vi "rsidr_core_global.vi"() -> ()   [LabVIEW 2015, in "Rohde&Schwarz CMXP NR FR2 Measurement.lvlib"] (continued)
s955, s956, s957, s958, s959, s960, s961, s962, s963, s964, s965, s966, s967, s968, s969, s970, s971, s972, s973, s974, s975, s976, s977, s978, s979, s980, s981, s982, s983, s984, s985, s986, s987, s988, s989, s990, s991, s992, s993, s994, s995, s996, s997, s998, s999, s1000\r\n\nRemote-control command(s):\nCONFigure:NRMMw:MEAS<i>:LIST:SEGMent<no>:SEMask"}, {"Level"=4, "Class Only"=FALSE, "Identifier"="RSCMXPNRFR2M_ATTR_MULTI_EVAL_MEASUREMENT_LIST_SEGMENT_ACLR", "Descriptive Name"="Multi Eval Measurement List Segment ACLR", "Data Type"=enum."RawString", "Command"="CONF:NRMM:MEAS{instance}:LIST:SEGM{Segment}:ACLR", "Access"=enum."Read/Write", "Range Table"="", "Read Callback"="", "Write Callback"="", "Range Callback"="", "Check Callback"="", "Rngtable Callback"="", "Coerce Callback"="", "Supported Models"="", "Instrument Options"="", "Check Status Callback"="", "Flags"=0, "Help"="Defines settings for ACLR measurements in list mode for segment <no>.\n\nSyntax:\nCONFigure:NRMMw:MEAS<i>:LIST:SEGMent<no>:ACLR <ACLRstatistics>, <ACLRenable>\n\n<ACLRstatistics>\nStatistical length in slots\ninteger\nValid Values: 1 to 1000\n \n<ACLRenable>\nEnable or disable the measurement of ACLR results\nValid Values:\nOFF\nON\n\nAvailable Repeated Capabilities:\ninstance: i0, i1, i2, i3, i4, i5, i6, i7, i8, i9, i10, i11, i12, i13, i14, i15, i16, i17, i18, i19, i20, i21, i22, i23, i24, i25, i26, i27, i28, i29, i30, i31, i32\r\nSegment: s1, s2, s3, s4, s5, s6, s7, s8, s9, s10, s11, s12, s13, s14, s15, s16, s17, s18, s19, s20, s21, s22, s23, s24, s25, s26, s27, s28, s29, s30, s31, s32, s33, s34, s35, s36, s37, s38, s39, s40, s41, s42, s43, s44, s45, s46, s47, s48, s49, s50, s51, s52, s53, s54, s55, s56, s57, s58, s59, s60, s61, s62, s63, s64, s65, s66, s67, s68, s69, s70, s71, s72, s73, s74, s75, s76, s77, s78, s79, s80, s81, s82, s83, s84, s85, s86, s87, s88, s89, s90, s91, s92, s93, s94, s95, s96, s97, s98, s99, s100, s101, s102, s103, s104, s105, s106, s107, s108, s109, s110, s111, s112, s113, s114, s115, s116, s117, s118, s119, s120, s121, s122, s123, s124, s125, s126, s127, s128, s129, s130, s131, s132, s133, s134, s135, s136, s137, s138, s139, s140, s141, s142, s143, s144, s145, s146, s147, s148, s149, s150, s151, s152, s153, s154, s155, s156, s157, s158, s159, s160, s161, s162, s163, s164, s165, s166, s167, s168, s169, s170, s171, s172, s173, s174, s175, s176, s177, s178, s179, s180, s181, s182, s183, s184, s185, s186, s187, s188, s189, s190, s191, s192, s193, s194, s195, s196, s197, s198, s199, s200, s201, s202, s203, s204, s205, s206, s207, s208, s209, s210, s211, s212, s213, s214, s215, s216, s217, s218, s219, s220, s221, s222, s223, s224, s225, s226, s227, s228, s229, s230, s231, s232, s233, s234, s235, s236, s237, s238, s239, s240, s241, s242, s243, s244, s245, s246, s247, s248, s249, s250, s251, s252, s253, s254, s255, s256, s257, s258, s259, s260, s261, s262, s263, s264, s265, s266, s267, s268, s269, s270, s271, s272, s273, s274, s275, s276, s277, s278, s279, s280, s281, s282, s283, s284, s285, s286, s287, s288, s289, s290, s291, s292, s293, s294, s295, s296, s297, s298, s299, s300, s301, s302, s303, s304, s305, s306, s307, s308, s309, s310, s311, s312, s313, s314, s315, s316, s317, s318, s319, s320, s321, s322, s323, s324, s325, s326, s327, s328, s329, s330, s331, s332, s333, s334, s335, s336, s337, s338, s339, s340, s341, s342, s343, s344, s345, s346, s347, s348, s349, s350, s351, s352, s353, s354, s355, s356, s357, s358, s359, s360, s361, s362, s363, s364, s365, s366, s367, s368, s369, s370, s371, s372, s373, s374, s375, s376, s377, s378, s379, s380, s381, s382, s383, s384, s385, s386, s387, s388, s389, s390, s391, s392, s393, s394, s395, s396, s397, s398, s399, s400, s401, s402, s403, s404, s405, s406, s407, s408, s409, s410, s411, s412, s413, s414, s415, s416, s417, s418, s419, s420, s421, s422, s423, s424, s425, s426, s427, s428, s429, s430, s431, s432, s433, s434, s435, s436, s437, s438, s439, s440, s441, s442, s443, s444, s445, s446, s447, s448, s449, s450, s451, s452, s453, s454, s455, s456, s457, s458, s459, s460, s461, s462, s463, s464, s465, s466, s467, s468, s469, s470, s471, s472, s473, s474, s475, s476, s477, s478, s479, s480, s481, s482, s483, s484, s485, s486, s487, s488, s489, s490, s491, s492, s493, s494, s495, s496, s497, s498, s499, s500, s501, s502, s503, s504, s505, s506, s507, s508, s509, s510, s511, s512, s513, s514, s515, s516, s517, s518, s519, s520, s521, s522, s523, s524, s525, s526, s527, s528, s529, s530, s531, s532, s533, s534, s535, s536, s537, s538, s539, s540, s541, s542, s543, s544, s545, s546, s547, s548, s549, s550, s551, s552, s553, s554, s555, s556, s557, s558, s559, s560, s561, s562, s563, s564, s565, s566, s567, s568, s569, s570, s571, s572, s573, s574, s575, s576, s577, s578, s579, s580, s581, s582, s583, s584, s585, s586, s587, s588, s589, s590, s591, s592, s593, s594, s595, s596, s597, s598, s599, s600, s601, s602, s603, s604, s605, s606, s607, s608, s609, s610, s611, s612, s613, s614, s615, s616, s617, s618, s619, s620, s621, s622, s623, s624, s625, s626, s627, s628, s629, s630, s631, s632, s633, s634, s635, s636, s637, s638, s639, s640, s641, s642, s643, s644, s645, s646, s647, s648, s649, s650, s651, s652, s653, s654, s655, s656, s657, s658, s659, s660, s661, s662, s663, s664, s665, s666, s667, s668, s669, s670, s671, s672, s673, s674, s675, s676, s677, s678, s679, s680, s681, s682, s683, s684, s685, s686, s687, s688, s689, s690, s691, s692, s693, s694, s695, s696, s697, s698, s699, s700, s701, s702, s703, s704, s705, s706, s707, s708, s709, s710, s711, s712, s713, s714, s715, s716, s717, s718, s719, s720, s721, s722, s723, s724, s725, s726, s727, s728, s729, s730, s731, s732, s733, s734, s735, s736, s737, s738, s739, s740, s741, s742, s743, s744, s745, s746, s747, s748, s749, s750, s751, s752, s753, s754, s755, s756, s757, s758, s759, s760, s761, s762, s763, s764, s765, s766, s767, s768, s769, s770, s771, s772, s773, s774, s775, s776, s777, s778, s779, s780, s781, s782, s783, s784, s785, s786, s787, s788, s789, s790, s791, s792, s793, s794, s795, s796, s797, s798, s799, s800, s801, s802, s803, s804, s805, s806, s807, s808, s809, s810, s811, s812, s813, s814, s815, s816, s817, s818, s819, s820, s821, s822, s823, s824, s825, s826, s827, s828, s829, s830, s831, s832, s833, s834, s835, s836, s837, s838, s839, s840, s841, s842, s843, s844, s845, s846, s847, s848, s849, s850, s851, s852, s853, s854, s855, s856, s857, s858, s859, s860, s861, s862, s863, s864, s865, s866, s867, s868, s869, s870, s871, s872, s873, s874, s875, s876, s877, s878, s879, s880, s881, s882, s883, s884, s885, s886, s887, s888, s889, s890, s891, s892, s893, s894, s895, s896, s897, s898, s899, s900, s901, s902, s903, s904, s905, s906, s907, s908, s909, s910, s911, s912, s913, s914, s915, s916, s917, s918, s919, s920, s921, s922, s923, s924, s925, s926, s927, s928, s929, s930, s931, s932, s933, s934, s935, s936, s937, s938, s939, s940, s941, s942, s943, s944, s945, s946, s947, s948, s949, s950, s951, s952, s953, s954, s955, s956, s957, s958, s959, s960, s961, s962, s963, s964, s965, s966, s967, s968, s969, s970, s971, s972, s973, s974, s975, s976, s977, s978, s979, s980, s981, s982, s983, s984, s985, s986, s987, s988, s989, s990, s991, s992, s993, s994, s995, s996, s997, s998, s999, s1000\r\n\nRemote-control command(s):\nCONFigure:NRMMw:MEAS<i>:LIST:SEGMent<no>:ACLR"}, {"Level"=2, "Class Only"=TRUE, "Identifier"="", "Descriptive Name"="Trigger", "Data Type"=enum."ViInt32", "Command"="", "Access"=enum."Read Only", "Range Table"="", "Read Callback"="", "Write Callback"="", "Range Callback"="", "Check Callback"="", "Rngtable Callback"="", "Coerce Callback"="", "Supported Models"="", "Instrument Options"="", "Check Status Callback"="", "Flags"=0, "Help"="Trigger settings"}, {"Level"=3, "Class Only"=FALSE, "Identifier"="RSCMXPNRFR2M_ATTR_MULTI_EVAL_MEASUREMENT_TRIGGER_SOURCE", "Descriptive Name"="Multi Eval Measurement Trigger Source", "Data Type"=enum."ViString", "Command"="TRIG:NRMM:MEAS{instance}:MEV:SOUR", "Access"=enum."Read/Write", "Range Table"="", "Read Callback"="", "Write Callback"="", "Range Callback"="", "Check Callback"="", "Rngtable Callback"="", "Coerce Callback"="", "Supported Models"="", "Instrument Options"="", "Check Status Callback"="", "Flags"=0, "Help"="Selects the source of the trigger events. Some values are always available. You can query a list of all supported values via TRIGger:...:CATalog:SOURce?\n\nAvailable Repeated Capabilities:\ninstance: i0, i1, i2, i3, i4, i5, i6, i7, i8, i9, i10, i11, i12, i13, i14, i15, i16, i17, i18, i19, i20, i21, i22, i23, i24, i25, i26, i27, i28, i29, i30, i31, i32\r\n\nRemote-control command(s):\nTRIGger:NRMMw:MEAS<i>:MEValuation:SOURce"}, {"Level"=3, "Class Only"=FALSE, "Identifier"="RSCMXPNRFR2M_ATTR_MULTI_EVAL_MEASUREMENT_TRIGGER_SOURCE_CATALOG", "Descriptive Name"="Multi Eval Measurement Trigger Source Catalog", "Data Type"=enum."RawString", "Command"="TRIG:NRMM:MEAS{instance}:MEV:CAT:SOUR?", "Access"=enum."Read Only", "Range Table"="", "Read Callback"="", "Write Callback"="", "Range Callback"="", "Check Callback"="", "Rngtable Callback"="", "Coerce Callback"="", "Supported Models"="", "Instrument Options"="", "Check Status Callback"="", "Flags"=0, "Help"="Lists all trigger source values that can be set using TRIGger:NRMMw:MEAS<i>:MEValuation:SOURce. Comma-separated list of all supported values, one string per value.\n\nAvailable Repeated Capabilities:\ninstance: i0, i1, i2, i3, i4, i5, i6, i7, i8, i9, i10, i11, i12, i13, i14, i15, i16, i17, i18, i19, i20, i21, i22, i23, i24, i25, i26, i27, i28, i29, i30, i31, i32\r\n\nRemote-control command(s):\nTRIGger:NRMMw:MEAS<i>:MEValuation:CATalog:SOURce?"}, {"Level"=3, "Class Only"=FALSE, "Identifier"="RSCMXPNRFR2M_ATTR_MULTI_EVAL_MEASUREMENT_TRIGGER_SLOPE", "Descriptive Name"="Multi Eval Measurement Trigger Slope", "Data Type"=enum."ViInt32", "Command"="TRIG:NRMM:MEAS{instance}:MEV:SLOP", "Access"=enum."Read/Write", "Range Table"="rsCmxpNrFr2M_rngTrigSlope", "Read Callback"="", "Write Callback"="", "Range Callback"="", "Check Callback"="", "Rngtable Callback"="", "Coerce Callback"="", "Supported Models"="", "Instrument Options"="", "Check Status Callback"="", "Flags"=0, "Help"="Qualifies whether the trigger event is generated at the rising or at the falling edge of the trigger pulse (valid for external and power trigger sources).\n\nAvailable Repeated Capabilities:\ninstance: i0, i1, i2, i3, i4, i5, i6, i7, i8, i9, i10, i11, i12, i13, i14, i15, i16, i17, i18, i19, i20, i21, i22, i23, i24, i25, i26, i27, i28, i29, i30, i31, i32\r\n\nRemote-control command(s):\nTRIGger:NRMMw:MEAS<i>:MEValuation:SLOPe"}, {"Level"=3, "Class Only"=FALSE, "Identifier"="RSCMXPNRFR2M_ATTR_MULTI_EVAL_MEASUREMENT_TRIGGER_THRESHOLD", "Descriptive Name"="Multi Eval Measurement Trigger Threshold", "Data Type"=enum."ViReal64", "Command"="TRIG:NRMM:MEAS{instance}:MEV:THR", "Access"=enum."Read/Write", "Range Table"="rsCmxpNrFr2M_rngTrigThreshold", "Read Callback"="", "Write Callback"="", "Range Callback"="", "Check Callback"="", "Rngtable Callback"="", "Coerce Callback"="", "Supported Models"="", "Instrument Options"="", "Check Status Callback"="", "Flags"=0, "Help"="Defines the trigger threshold for power trigger sources.\n\nAvailable Repeated Capabilities:\ninstance: i0, i1, i2, i3, i4, i5, i6, i7, i8, i9, i10, i11, i12, i13, i14, i15, i16, i17, i18, i19, i20, i21, i22, i23, i24, i25, i26, i27, i28, i29, i30, i31, i32\r\n\nRemote-control command(s):\nTRIGger:NRMMw:MEAS<i>:MEValuation:THReshold"}, {"Level"=3, "Class Only"=FALSE, "Identifier"="RSCMXPNRFR2M_ATTR_MULTI_EVAL_MEASUREMENT_TRIGGER_DELAY", "Descriptive Name"="Multi Eval Measurement Trigger Delay", "Data Type"=enum."ViReal64", "Command"="TRIG:NRMM:MEAS{instance}:MEV:DEL", "Access"=enum."Read/Write", "Range Table"="rsCmxpNrFr2M_rngMultiEvalMeasurementTriggerDelay", "Read Callback"="", "Write Callback"="", "Range Callback"="", "Check Callback"="", "Rngtable Callback"="", "Coerce Callback"="", "Supported Models"="", "Instrument Options"="", "Check Status Callback"="", "Flags"=0, "Help"="Defines a time delaying the start of the measurement relative to the trigger event. This setting has no influence on free run measurements.\n\nAvailable Repeated Capabilities:\ninstance: i0, i1, i2, i3, i4, i5, i6, i7, i8, i9, i10, i11, i12, i13, i14, i15, i16, i17, i18, i19, i20, i21, i22, i23, i24, i25, i26, i27, i28, i29, i30, i31, i32\r\n\nRemote-control command(s):\nTRIGger:NRMMw:MEAS<i>:MEValuation:DELay"}, {"Level"=3, "Class Only"=FALSE, "Identifier"="RSCMXPNRFR2M_ATTR_MULTI_EVAL_MEASUREMENT_TRIGGER_TIMEOUT_ENABLED", "Descriptive Name"="Multi Eval Measurement Trigger Timeout Enabled", "Data Type"=enum."ViBoolean", "Command"="TRIG:NRMM:MEAS{instance}:MEV:TOUT", "Access"=enum."Write Only", "Range Table"="", "Read Callback"="", "Write Callback"="", "Range Callback"="", "Check Callback"="", "Rngtable Callback"="", "Coerce Callback"="", "Supported Models"="", "Instrument Options"="", "Check Status Callback"="", "Flags"=0, "Help"="Enables/disables trigger timeout.\n\nAvailable Repeated Capabilities:\ninstance: i0, i1, i2, i3, i4, i5, i6, i7, i8, i9, i10, i11, i12, i13, i14, i15, i16, i17, i18, i19, i20, i21, i22, i23, i24, i25, i26, i27, i28, i29, i30, i31, i32\r\n\nRemote-control command(s):\nTRIGger:NRMMw:MEAS<i>:MEValuation:TOUT"}, {"Level"=3, "Class Only"=FALSE, "Identifier"="RSCMXPNRFR2M_ATTR_MULTI_EVAL_MEASUREMENT_TRIGGER_TIMEOUT", "Descriptive Name"="Multi Eval Measurement Trigger Timeout", "Data Type"=enum."ViReal64", "Command"="TRIG:NRMM:MEAS{instance}:MEV:TOUT", "Access"=enum."Read/Write", "Range Table"="rsCmxpNrFr2M_rngTriggerTimeout", "Read Callback"="", "Write Callback"="", "Range Callback"="", "Check Callback"="", "Rngtable Callback"="", "Coerce Callback"="", "Supported Models"="", "Instrument Options"="", "Check Status Callback"="", "Flags"=0, "Help"="Selects the maximum time that the measurement waits for a trigger event before it stops in remote control mode or indicates a trigger timeout in manual operation mode. This setting has no influence on 'Free Run' measurements.\n\nAvailable Repeated Capabilities:\ninstance: i0, i1, i2, i3, i4, i5, i6, i7, i8, i9, i10, i11, i12, i13, i14, i15, i16, i17, i18, i19, i20, i21, i22, i23, i24, i25, i26, i27, i28, i29, i30, i31, i32\r\n\nRemote-control command(s):\nTRIGger:NRMMw:MEAS<i>:MEValuation:TOUT"}, {"Level"=3, "Class Only"=FALSE, "Identifier"="RSCMXPNRFR2M_ATTR_MULTI_EVAL_MEASUREMENT_MINIMUM_TRIGGER_GAP", "Descriptive Name"="Multi Eval Measurement Minimum Trigger Gap", "Data Type"=enum."ViReal64", "Command"="TRIG:NRMM:MEAS{instance}:MEV:MGAP", "Access"=enum."Read/Write", "Range Table"="rsCmxpNrFr2M_rngMultiEvalMeasurementMinimumTriggerGap", "Read Callback"="", "Write Callback"="", "Range Callback"="", "Check Callback"="", "Rngtable Callback"="", "Coerce Callback"="", "Supported Models"="", "Instrument Options"="", "Check Status Callback"="", "Flags"=0, "Help"="Sets a minimum time during which the IF signal must be below the trigger threshold before the trigger is armed so that an IF power trigger event can be generated.\n\nAvailable Repeated Capabilities:\ninstance: i0, i1, i2, i3, i4, i5, i6, i7, i8, i9, i10, i11, i12, i13, i14, i15, i16, i17, i18, i19, i20, i21, i22, i23, i24, i25, i26, i27, i28, i29, i30, i31, i32\r\n\nRemote-control command(s):\nTRIGger:NRMMw:MEAS<i>:MEValuation:MGAP"}, {"Level"=2, "Class Only"=TRUE, "Identifier"="", "Descriptive Name"="Limits", "Data Type"=enum."ViInt32", "Command"="", "Access"=enum."Read Only", "Range Table"="", "Read Callback"="", "Write Callback"="", "Range Callback"="", "Check Callback"="", "Rngtable Callback"="", "Coerce Callback"="", "Supported Models"="", "Instrument Options"="", "Check Status Callback"="", "Flags"=0, "Help"="Multi Evaluation measurement limits attributes."}, {"Level"=3, "Class Only"=TRUE, "Identifier"="", "Descriptive Name"="Modulation", "Data Type"=enum."ViInt32", "Command"="", "Access"=enum."Read Only", "Range Table"="", "Read Callback"="", "Write Callback"="", "Range Callback"="", "Check Callback"="", "Rngtable Callback"="", "Coerce Callback"="", "Supported Models"="", "Instrument Options"="", "Check Status Callback"="", "Flags"=0, "Help"="Modulation attributes."}, {"Level"=4, "Class Only"=TRUE, "Identifier"="", "Descriptive Name"="Pi/2-BPSK", "Data Type"=enum."ViInt32", "Command"="", "Access"=enum."Read Only", "Range Table"="", "Read Callback"="", "Write Callback"="", "Range Callback"="", "Check Callback"="", "Rngtable Callback"="", "Coerce Callback"="", "Supported Models"="", "Instrument Options"="", "Check Status Callback"="", "Flags"=0, "Help"="Define limits for results which characterize the modulation accuracy of signals with modulation scheme Pi/2-BPSK."}, {"Level"=5, "Class Only"=FALSE, "Identifier"="RSCMXPNRFR2M_ATTR_MULTI_EVAL_MEASUREMENT_LIMIT_PHBPSK_EVM", "Descriptive Name"="Multi Eval Measurement Limit PHBPSK EVM", "Data Type"=enum."RawString", "Command"="CONF:NRMM:MEAS{instance}:MEV:LIM:PHBP:EVM", "Access"=enum."Read/Write", "Range Table"="", "Read Callback"="", "Write Callback"="", "Range Callback"="", "Check Callback"="", "Rngtable Callback"="", "Coerce Callback"="", "Supported Models"="", "Instrument Options"="", "Check Status Callback"="", "Flags"=0, "Help"="Defines upper limits for the RMS and peak values of the error vector magnitude (EVM) for Pi/2-BPSK.\n\nSyntax:\nCONFigure:NRMMw:MEAS<i>:MEValuation:LIMit:PHBPsk:EVMagnitude <RMS>, <Peak>\n\n<RMS>\nnumeric | ON | OFF\nValid Values:\n0 % to 100 %\nOFF\nON\n  \n<Peak>\nnumeric | ON | OFF\nValid Values:\n0 % to 100 %\nOFF\nON\n\nAvailable Repeated Capabilities:\ninstance: i0, i1, i2, i3, i4, i5, i6, i7, i8, i9, i10, i11, i12, i13, i14, i15, i16, i17, i18, i19, i20, i21, i22, i23, i24, i25, i26, i27, i28, i29, i30, i31, i32\r\n\nRemote-control command(s):\nCONFigure:NRMMw:MEAS<i>:MEValuation:LIMit:PHBPsk:EVMagnitude"}, {"Level"=5, "Class Only"=FALSE, "Identifier"="RSCMXPNRFR2M_ATTR_MULTI_EVAL_MEASUREMENT_LIMIT_PHBPSK_MERR", "Descriptive Name"="Multi Eval Measurement Limit PHBPSK MERR", "Data Type"=enum."RawString", "Command"="CONF:NRMM:MEAS{instance}:MEV:LIM:PHBP:MERR", "Access"=enum."Read/Write", "Range Table"="", "Read Callback"="", "Write Callback"="", "Range Callback"="", "Check Callback"="", "Rngtable Callback"="", "Coerce Callback"="", "Supported Models"="", "Instrument Options"="", "Check Status Callback"="", "Flags"=0, "Help"="Defines upper limits for the RMS and peak values of the magnitude error (MERR)  for Pi/2-BPSK.\n\nSyntax:\nCONFigure:NRMMw:MEAS<i>:MEValuation:LIMit:PHBPsk:MERRor <RMS>, <Peak>\n\n<RMS>\nnumeric | ON | OFF\nValid Values:\n0 % to 100 %\nOFF\nON\n  \n<Peak>\nnumeric | ON | OFF\nValid Values:\n0 % to 100 %\nOFF\nON\n\nAvailable Repeated Capabilities:\ninstance: i0, i1, i2, i3, i4, i5, i6, i7, i8, i9, i10, i11, i12, i13, i14, i15, i16, i17, i18, i19, i20, i21, i22, i23, i24, i25, i26, i27, i28, i29, i30, i31, i32\r\n\nRemote-control command(s):\nCONFigure:NRMMw:MEAS<i>:MEValuation:LIMit:PHBPsk:MERRor"}, {"Level"=5, "Class Only"=FALSE, "Identifier"="RSCMXPNRFR2M_ATTR_MULTI_EVAL_MEASUREMENT_LIMIT_PHBPSK_PERR", "Descriptive Name"="Multi Eval Measurement Limit PHBPSK PERR", "Data Type"=enum."RawString", "Command"="CONF:NRMM:MEAS{instance}:MEV:LIM:PHBP:PERR", "Access"=enum."Read/Write", "Range Table"="", "Read Callback"="", "Write Callback"="", "Range Callback"="", "Check Callback"="", "Rngtable Callback"="", "Coerce Callback"="", "Supported Models"="", "Instrument Options"="", "Check Status Callback"="", "Flags"=0, "Help"="Defines upper limits for the RMS and peak values of the phase error (PERR)  for Pi/2-BPSK.\n\nSyntax:\nCONFigure:NRMMw:MEAS<i>:MEValuation:LIMit:PHBPsk:PERRor <RMS>, <Peak>\n\n<RMS>\nnumeric | ON | OFF\nValid Values:\n0 % to 100 %\nOFF\nON\n  \n<Peak>\nnumeric | ON | OFF\nValid Values:\n0 % to 100 %\nOFF\nON\n\nAvailable Repeated Capabilities:\ninstance: i0, i1, i2, i3, i4, i5, i6, i7, i8, i9, i10, i11, i12, i13, i14, i15, i16, i17, i18, i19, i20, i21, i22, i23, i24, i25, i26, i27, i28, i29, i30, i31, i32\r\n\nRemote-control command(s):\nCONFigure:NRMMw:MEAS<i>:MEValuation:LIMit:PHBPsk:PERRor"}, {"Level"=5, "Class Only"=FALSE, "Identifier"="RSCMXPNRFR2M_ATTR_MULTI_EVAL_MEASUREMENT_LIMIT_PHBPSK_FERR", "Descriptive Name"="Multi Eval Measurement Limit PHBPSK FERR", "Data Type"=enum."RawString", "Command"="CONF:NRMM:MEAS{instance}:MEV:LIM:PHBP:FERR", "Access"=enum."Read/Write", "Range Table"="", "Read Callback"="", "Write Callback"="", "Range Callback"="", "Check Callback"="", "Rngtable Callback"="", "Coerce Callback"="", "Supported Models"="", "Instrument Options"="", "Check Status Callback"="", "Flags"=0, "Help"="Defines an upper limit for the carrier frequency error (Pi/2-BPSK modulation).\n\nSyntax:\nCONFigure:NRMMw:MEAS<i>:MEValuation:LIMit:PHBPsk:FERRor <FrequencyError>\n\n<FrequencyError>\nnumeric | ON | OFF\nValid Values:\n0 to 1 ppm\nOFF\nON\n\nAvailable Repeated Capabilities:\ninstance: i0, i1, i2, i3, i4, i5, i6, i7, i8, i9, i10, i11, i12, i13, i14, i15, i16, i17, i18, i19, i20, i21, i22, i23, i24, i25, i26, i27, i28, i29, i30, i31, i32\r\n\nRemote-control command(s):\nCONFigure:NRMMw:MEAS<i>:MEValuation:LIMit:PHBPsk:FERRor"}, {"Level"=5, "Class Only"=FALSE, "Identifier"="RSCMXPNRFR2M_ATTR_MULTI_EVAL_MEASUREMENT_LIMIT_PHBPSK_IQ_OFFSET", "Descriptive Name"="Multi Eval Measurement Limit PHBPSK IQ Offset", "Data Type"=enum."RawString", "Command"="CONF:NRMM:MEAS{instance}:MEV:LIM:PHBP:IQOF", "Access"=enum."Read/Write", "Range Table"="", "Read Callback"="", "Write Callback"="", "Range Callback"="", "Check Callback"="", "Rngtable Callback"="", "Coerce Callback"="", "Supported Models"="", "Instrument Options"="", "Check Status Callback"="", "Flags"=0, "Help"="Defines upper limits for the I/Q origin offset (Pi/2-BPSK modulation). Two different I/Q origin offset limits can be set for two TX power ranges.\n\nSyntax:\nCONFigure:NRMMw:MEAS<i>:MEValuation:LIMit:PHBPsk:IQOFfset <Enable>, <Offset0>, <Offset1>\n\n<Enable>\nValid Values:\nOFF: disables the limit check\nON: enables the limit check\n\n<Offset0>\nI/Q origin offset limit for TX power > 0 dBm\nnumeric\nValid Values: -256 dBc to 256 dBc\n\n<Offset1>\nI/Q origin offset limit for TX power  0 dBm\nnumeric\nValid Values: -256 dBc to 256 dBc\n\nAvailable Repeated Capabilities:\ninstance: i0, i1, i2, i3, i4, i5, i6, i7, i8, i9, i10, i11, i12, i13, i14, i15, i16, i17, i18, i19, i20, i21, i22, i23, i24, i25, i26, i27, i28, i29, i30, i31, i32\r\n\nRemote-control command(s):\nCONFigure:NRMMw:MEAS<i>:MEValuation:LIMit:PHBPsk:IQOFfset"}, {"Level"=5, "Class Only"=FALSE, "Identifier"="RSCMXPNRFR2M_ATTR_MULTI_EVAL_MEASUREMENT_LIMIT_PHBPSK_INBAND_EMISSION", "Descriptive Name"="Multi Eval Measurement Limit PHBPSK Inband Emission", "Data Type"=enum."RawString", "Command"="CONF:NRMM:MEAS{instance}:MEV:LIM:PHBP:IBE", "Access"=enum."Read/Write", "Range Table"="", "Read Callback"="", "Write Callback"="", "Range Callback"="", "Check Callback"="", "Rngtable Callback"="", "Coerce Callback"="", "Supported Models"="", "Instrument Options"="", "Check Status Callback"="", "Flags"=0, "Help"="Defines parameters used for calculation of an upper limit for the inband emission (Pi/2-BPSK modulation).\n\nSyntax:\nCONFigure:NRMMw:MEAS<i>:MEValuation:LIMit:PHBPsk:IQOFfset <Enable>, <Offset0>, <Offset1>\n\n<Enable>\nValid Values:\nOFF: disables the limit check\nON: enables the limit check\n\n<Minimum>\nnumeric\nValid Values: -256 dB to 256 dB\n\n<EVM>\nnumeric\nValid Values: 0 % to 100 %\n\n<RBPower>\nnumeric\nValid Values: -256 dBm to 256 dBm\n\n<IQImageLesser>\nIQ image for low TX power range\nnumeric\nValid Values: -256 dB to 256 dB\n \n<IQImageGreater>\nIQ image for high TX power range\nnumeric\nValid Values: -256 dB  to  256 dB\n\nAvailable Repeated Capabilities:\ninstance: i0, i1, i2, i3, i4, i5, i6, i7, i8, i9, i10, i11, i12, i13, i14, i15, i16, i17, i18, i19, i20, i21, i22, i23, i24, i25, i26, i27, i28, i29, i30, i31, i32\r\n\nRemote-control command(s):\nCONFigure:NRMMw:MEAS<i>:MEValuation:LIMit:PHBPsk:IBE"}, {"Level"=5, "Class Only"=FALSE, "Identifier"="RSCMXPNRFR2M_ATTR_MULTI_EVAL_MEASUREMENT_LIMIT_PHBPSK_INBAND_EMISSION_IQ_OFFSET", "Descriptive Name"="Multi Eval Measurement Limit PHBPSK Inband Emission IQ Offset", "Data Type"=enum."RawString", "Command"="CONF:NRMM:MEAS{instance}:MEV:LIM:PHBP:IBE:IQOF", "Access"=enum."Read/Write", "Range Table"="", "Read Callback"="", "Write Callback"="", "Range Callback"="", "Check Callback"="", "Rngtable Callback"="", "Coerce Callback"="", "Supported Models"="", "Instrument Options"="", "Check Status Callback"="", "Flags"=0, "Help"="Defines I/Q origin offset values used for calculation of an upper limit for the inband emission, for Pi/2-BPSK modulation. Two different values can be set for two TX power ranges.\n\nSyntax:\nCONFigure:NRMMw:MEAS<i>:MEValuation:LIMit:PHBPsk:IBE:IQOFfset <Offset0>, <Offset1>\n\n<Offset0>\nI/Q origin offset limit for TX power > 0 dBm\nnumeric\nValid Values: -256 dBc to 256 dBc\n\n<Offset1>\nI/Q origin offset limit for TX power  0 dBm\nnumeric\nValid Values: -256 dBc to 256 dBc\n\nAvailable Repeated Capabilities:\ninstance: i0, i1, i2, i3, i4, i5, i6, i7, i8, i9, i10, i11, i12, i13, i14, i15, i16, i17, i18, i19, i20, i21, i22, i23, i24, i25, i26, i27, i28, i29, i30, i31, i32\r\n\nRemote-control command(s):\nCONFigure:NRMMw:MEAS<i>:MEValuation:LIMit:PHBPsk:IBE:IQOFfset"}, {"Level"=5, "Class Only"=FALSE, "Identifier"="RSCMXPNRFR2M_ATTR_MULTI_EVAL_MEASUREMENT_LIMIT_PHBPSK_EQUALIZER_SPECTRUM_FLATNESS", "Descriptive Name"="Multi Eval Measurement Limit PHBPSK Equalizer Spectrum Flatness", "Data Type"=enum."RawString", "Command"="CONF:NRMM:MEAS{instance}:MEV:LIM:PHBP:ESFL", "Access"=enum."Read/Write", "Range Table"="", "Read Callback"="", "Write Callback"="", "Range Callback"="", "Check Callback"="", "Rngtable Callback"="", "Coerce Callback"="", "Supported Models"="", "Instrument Options"="", "Check Status Callback"="", "Flags"=0, "Help"="Defines limits for the equalizer spectrum flatness (Pi/2-BPSK modulation).\n\nSyntax:\nCONFigure:NRMMw:MEAS<i>:MEValuation:LIMit:PHBPsk:IQOFfset <Enable>, <Offset0>, <Offset1>\n\n<Enable>\nValid Values:\nOFF: disables the limit check\nON: enables the limit check\n\n<Range1>\nUpper limit for max(range 1) - min(range 1)\nnumeric\nValid Values: -256 dBpp to 256 dBpp \n\n<Range2>\nUpper limit for max(range 2) - min(range 2)\nnumeric\nValid Values: -256 dBpp to 256 dBpp \n\n<Max1Min2>\nUpper limit for max(range 1) - min(range 2)\nnumeric\nValid Values: -256 dB to 256 dB \n\n<Max2Min1>\nUpper limit for max(range 2) - min(range 1)\nnumeric\nValid Values: -256 dB to 256 dB\n\nAvailable Repeated Capabilities:\ninstance: i0, i1, i2, i3, i4, i5, i6, i7, i8, i9, i10, i11, i12, i13, i14, i15, i16, i17, i18, i19, i20, i21, i22, i23, i24, i25, i26, i27, i28, i29, i30, i31, i32\r\n\nRemote-control command(s):\nCONFigure:NRMMw:MEAS<i>:MEValuation:LIMit:PHBPsk:ESFLatness"}, {"Level"=4, "Class Only"=TRUE, "Identifier"="", "Descriptive Name"="QPSK", "Data Type"=enum."ViInt32", "Command"="", "Access"=enum."Read Only", "Range Table"="", "Read Callback"="", "Write Callback"="", "Range Callback"="", "Check Callback"="", "Rngtable Callback"="", "Coerce Callback"="", "Supported Models"="", "Instrument Options"="", "Check Status Callback"="", "Flags"=0, "Help"="QPSK modulation limits definition."}, {"Level"=5, "Class Only"=FALSE, "Identifier"="RSCMXPNRFR2M_ATTR_MULTI_EVAL_MEASUREMENT_LIMIT_QPSK_EVM", "Descriptive Name"="Multi Eval Measurement Limit QPSK EVM", "Data Type"=enum."RawString", "Command"="CONF:NRMM:MEAS{instance}:MEV:LIM:QPSK:EVM", "Access"=enum."Read/Write", "Range Table"="", "Read Callback"="", "Write Callback"="", "Range Callback"="", "Check Callback"="", "Rngtable Callback"="", "Coerce Callback"="", "Supported Models"="", "Instrument Options"="", "Check Status Callback"="", "Flags"=0, "Help"="Defines upper limits for the RMS and peak values of the error vector magnitude (EVM) for QPSK.\n\nSyntax:\nCONFigure:NRMMw:MEAS<i>:MEValuation:LIMit:QPSK:EVMagnitude <RMS>, <Peak>\n\n<RMS>\nnumeric | ON | OFF\nValid Values:\n0 % to 100 %\nOFF\nON\n  \n<Peak>\nnumeric | ON | OFF\nValid Values:\n0 % to 100 %\nOFF\nON\n\nAvailable Repeated Capabilities:\ninstance: i0, i1, i2, i3, i4, i5, i6, i7, i8, i9, i10, i11, i12, i13, i14, i15, i16, i17, i18, i19, i20, i21, i22, i23, i24, i25, i26, i27, i28, i29, i30, i31, i32\r\n\nRemote-control command(s):\nCONFigure:NRMMw:MEAS<i>:MEValuation:LIMit:QPSK:EVMagnitude"}, {"Level"=5, "Class Only"=FALSE, "Identifier"="RSCMXPNRFR2M_ATTR_MULTI_EVAL_MEASUREMENT_LIMIT_QPSK_MERR", "Descriptive Name"="Multi Eval Measurement Limit QPSK MERR", "Data Type"=enum."RawString", "Command"="CONF:NRMM:MEAS{instance}:MEV:LIM:QPSK:MERR", "Access"=enum."Read/Write", "Range Table"="", "Read Callback"="", "Write Callback"="", "Range Callback"="", "Check Callback"="", "Rngtable Callback"="", "Coerce Callback"="", "Supported Models"="", "Instrument Options"="", "Check Status Callback"="", "Flags"=0, "Help"="Defines upper limits for the RMS and peak values of the magnitude error (MERR)  for QPSK.\n\nSyntax:\nCONFigure:NRMMw:MEAS<i>:MEValuation:LIMit:QPSK:MERRor <RMS>, <Peak>\n\n<RMS>\nnumeric | ON | OFF\nValid Values:\n0 % to 100 %\nOFF\nON\n  \n<Peak>\nnumeric | ON | OFF\nValid Values:\n0 % to 100 %\nOFF\nON\n\nAvailable Repeated Capabilities:\ninstance: i0, i1, i2, i3, i4, i5, i6, i7, i8, i9, i10, i11, i12, i13, i14, i15, i16, i17, i18, i19, i20, i21, i22, i23, i24, i25, i26, i27, i28, i29, i30, i31, i32\r\n\nRemote-control command(s):\nCONFigure:NRMMw:MEAS<i>:MEValuation:LIMit:QPSK:MERRor"}, {"Level"=5, "Class Only"=FALSE, "Identifier"="RSCMXPNRFR2M_ATTR_MULTI_EVAL_MEASUREMENT_LIMIT_QPSK_PERR", "Descriptive Name"="Multi Eval Measurement Limit QPSK PERR", "Data Type"=enum."RawString", "Command"="CONF:NRMM:MEAS{instance}:MEV:LIM:QPSK:PERR", "Access"=enum."Read/Write", "Range Table"="", "Read Callback"="", "Write Callback"="", "Range Callback"="", "Check Callback"="", "Rngtable Callback"="", "Coerce Callback"="", "Supported Models"="", "Instrument Options"="", "Check Status Callback"="", "Flags"=0, "Help"="Defines upper limits for the RMS and peak values of the phase error (PERR)  for QPSK.\n\nSyntax:\nCONFigure:NRMMw:MEAS<i>:MEValuation:LIMit:QPSK:PERRor <RMS>, <Peak>\n\n<RMS>\nnumeric | ON | OFF\nValid Values:\n0 % to 100 %\nOFF\nON\n  \n<Peak>\nnumeric | ON | OFF\nValid Values:\n0 % to 100 %\nOFF\nON\n\nAvailable Repeated Capabilities:\ninstance: i0, i1, i2, i3, i4, i5, i6, i7, i8, i9, i10, i11, i12, i13, i14, i15, i16, i17, i18, i19, i20, i21, i22, i23, i24, i25, i26, i27, i28, i29, i30, i31, i32\r\n\nRemote-control command(s):\nCONFigure:NRMMw:MEAS<i>:MEValuation:LIMit:QPSK:PERRor"}, {"Level"=5, "Class Only"=FALSE, "Identifier"="RSCMXPNRFR2M_ATTR_MULTI_EVAL_MEASUREMENT_LIMIT_QPSK_FERR", "Descriptive Name"="Multi Eval Measurement Limit QPSK FERR", "Data Type"=enum."RawString", "Command"="CONF:NRMM:MEAS{instance}:MEV:LIM:QPSK:FERR", "Access"=enum."Read/Write", "Range Table"="", "Read Callback"="", "Write Callback"="", "Range Callback"="", "Check Callback"="", "Rngtable Callback"="", "Coerce Callback"="", "Supported Models"="", "Instrument Options"="", "Check Status Callback"="", "Flags"=0, "Help"="Defines an upper limit for the carrier frequency error (QPSK modulation).\n\nSyntax:\nCONFigure:NRMMw:MEAS<i>:MEValuation:LIMit:PHBPsk:FERRor <FrequencyError>\n\n<FrequencyError>\nnumeric | ON | OFF\nValid Values:\n0 to 1 ppm\nOFF\nON\n\nAvailable Repeated Capabilities:\ninstance: i0, i1, i2, i3, i4, i5, i6, i7, i8, i9, i10, i11, i12, i13, i14, i15, i16, i17, i18, i19, i20, i21, i22, i23, i24, i25, i26, i27, i28, i29, i30, i31, i32\r\n\nRemote-control command(s):\nCONFigure:NRMMw:MEAS<i>:MEValuation:LIMit:QPSK:FERRor"}, {"Level"=5, "Class Only"=FALSE, "Identifier"="RSCMXPNRFR2M_ATTR_MULTI_EVAL_MEASUREMENT_LIMIT_QPSK_IQ_OFFSET", "Descriptive Name"="Multi Eval Measurement Limit QPSK IQ Offset", "Data Type"=enum."RawString", "Command"="CONF:NRMM:MEAS{instance}:MEV:LIM:QPSK:IQOF", "Access"=enum."Read/Write", "Range Table"="", "Read Callback"="", "Write Callback"="", "Range Callback"="", "Check Callback"="", "Rngtable Callback"="", "Coerce Callback"="", "Supported Models"="", "Instrument Options"="", "Check Status Callback"="", "Flags"=0, "Help"="Defines upper limits for the I/Q origin offset (QPSK modulation). Two different I/Q origin offset limits can be set for two TX power ranges.\n\nSyntax:\nCONFigure:NRMMw:MEAS<i>:MEValuation:LIMit:QPSK:IQOFfset <Enable>, <Offset0>, <Offset1>\n\n<Enable>\nValid Values:\nOFF: disables the limit check\nON: enables the limit check\n\n<Offset0>\nI/Q origin offset limit for TX power > 0 dBm\nnumeric\nValid Values: -256 dBc to 256 dBc\n\n<Offset1>\nI/Q origin offset limit for TX power  0 dBm\nnumeric\nValid Values: -256 dBc to 256 dBc\n\nAvailable Repeated Capabilities:\ninstance: i0, i1, i2, i3, i4, i5, i6, i7, i8, i9, i10, i11, i12, i13, i14, i15, i16, i17, i18, i19, i20, i21, i22, i23, i24, i25, i26, i27, i28, i29, i30, i31, i32\r\n\nRemote-control command(s):\nCONFigure:NRMMw:MEAS<i>:MEValuation:LIMit:QPSK:IQOFfset"}, {"Level"=5, "Class Only"=FALSE, "Identifier"="RSCMXPNRFR2M_ATTR_MULTI_EVAL_MEASUREMENT_LIMIT_QPSK_INBAND_EMISSION", "Descriptive Name"="Multi Eval Measurement Limit QPSK Inband Emission", "Data Type"=enum."RawString", "Command"="CONF:NRMM:MEAS{instance}:MEV:LIM:QPSK:IBE", "Access"=enum."Read/Write", "Range Table"="", "Read Callback"="", "Write Callback"="", "Range Callback"="", "Check Callback"="", "Rngtable Callback"="", "Coerce Callback"="", "Supported Models"="", "Instrument Options"="", "Check Status Callback"="", "Flags"=0, "Help"="Defines parameters used for calculation of an upper limit for the inband emission (QPSK modulation).\n\nSyntax:\nCONFigure:NRMMw:MEAS<i>:MEValuation:LIMit:QPSK:IQOFfset <Enable>, <Offset0>, <Offset1>\n\n<Enable>\nValid Values:\nOFF: disables the limit check\nON: enables the limit check\n\n<Minimum>\nnumeric\nValid Values: -256 dB to 256 dB\n\n<EVM>\nnumeric\nValid Values: 0 % to 100 %\n\n<RBPower>\nnumeric\nValid Values: -256 dBm to 256 dBm\n\n<IQImageLesser>\nIQ image for low TX power range\nnumeric\nValid Values: -256 dB to 256 dB\n \n<IQImageGreater>\nIQ image for high TX power range\nnumeric\nValid Values: -256 dB  to  256 dB\n\nAvailable Repeated Capabilities:\ninstance: i0, i1, i2, i3, i4, i5, i6, i7, i8, i9, i10, i11, i12, i13, i14, i15, i16, i17, i18, i19, i20, i21, i22, i23, i24, i25, i26, i27, i28, i29, i30, i31, i32\r\n\nRemote-control command(s):\nCONFigure:NRMMw:MEAS<i>:MEValuation:LIMit:QPSK:IBE"}, {"Level"=5, "Class Only"=FALSE, "Identifier"="RSCMXPNRFR2M_ATTR_MULTI_EVAL_MEASUREMENT_LIMIT_QPSK_INBAND_EMISSION_IQ_OFFSET", "Descriptive Name"="Multi Eval Measurement Limit QPSK Inband Emission IQ Offset", "Data Type"=enum."RawString", "Command"="CONF:NRMM:MEAS{instance}:MEV:LIM:QPSK:IBE:IQOF", "Access"=enum."Read/Write", "Range Table"="", "Read Callback"="", "Write Callback"="", "Range Callback"="", "Check Callback"="", "Rngtable Callback"="", "Coerce Callback"="", "Supported Models"="", "Instrument Options"="", "Check Status Callback"="", "Flags"=0, "Help"="Defines I/Q origin offset values used for calculation of an upper limit for the inband emission, for QPSK modulation. Two different values can be set for two TX power ranges.\n\nSyntax:\nCONFigure:NRMMw:MEAS<i>:MEValuation:LIMit:QPSK:IBE:IQOFfset <Offset0>, <Offset1>\n\n<Offset0>\nI/Q origin offset limit for TX power > 0 dBm\nnumeric\nValid Values: -256 dBc to 256 dBc\n\n<Offset1>\nI/Q origin offset limit for TX power  0 dBm\nnumeric\nValid Values: -256 dBc to 256 dBc\n\nAvailable Repeated Capabilities:\ninstance: i0, i1, i2, i3, i4, i5, i6, i7, i8, i9, i10, i11, i12, i13, i14, i15, i16, i17, i18, i19, i20, i21, i22, i23, i24, i25, i26, i27, i28, i29, i30, i31, i32\r\n\nRemote-control command(s):\nCONFigure:NRMMw:MEAS<i>:MEValuation:LIMit:QPSK:IBE:IQOFfset"}, {"Level"=5, "Class Only"=FALSE, "Identifier"="RSCMXPNRFR2M_ATTR_MULTI_EVAL_MEASUREMENT_LIMIT_QPSK_EQUALIZER_SPECTRUM_FLATNESS", "Descriptive Name"="Multi Eval Measurement Limit QPSK Equalizer Spectrum Flatness", "Data Type"=enum."RawString", "Command"="CONF:NRMM:MEAS{instance}:MEV:LIM:QPSK:ESFL", "Access"=enum."Read/Write", "Range Table"="", "Read Callback"="", "Write Callback"="", "Range Callback"="", "Check Callback"="", "Rngtable Callback"="", "Coerce Callback"="", "Supported Models"="", "Instrument Options"="", "Check Status Callback"="", "Flags"=0, "Help"="Defines limits for the equalizer spectrum flatness (QPSK modulation).\n\nSyntax:\nCONFigure:NRMMw:MEAS<i>:MEValuation:LIMit:QPSK:IQOFfset <Enable>, <Offset0>, <Offset1>\n\n<Enable>\nValid Values:\nOFF: disables the limit check\nON: enables the limit check\n\n<Range1>\nUpper limit for max(range 1) - min(range 1)\nnumeric\nValid Values: -256 dBpp to 256 dBpp \n\n<Range2>\nUpper limit for max(range 2) - min(range 2)\nnumeric\nValid Values: -256 dBpp to 256 dBpp \n\n<Max1Min2>\nUpper limit for max(range 1) - min(range 2)\nnumeric\nValid Values: -256 dB to 256 dB \n\n<Max2Min1>\nUpper limit for max(range 2) - min(range 1)\nnumeric\nValid Values: -256 dB to 256 dB\n\nAvailable Repeated Capabilities:\ninstance: i0, i1, i2, i3, i4, i5, i6, i7, i8, i9, i10, i11, i12, i13, i14, i15, i16, i17, i18, i19, i20, i21, i22, i23, i24, i25, i26, i27, i28, i29, i30, i31, i32\r\n\nRemote-control command(s):\nCONFigure:NRMMw:MEAS<i>:MEValuation:LIMit:QPSK:ESFLatness"}, {"Level"=4, "Class Only"=TRUE, "Identifier"="", "Descriptive Name"="QAM", "Data Type"=enum."ViInt32", "Command"="", "Access"=enum."Read Only", "Range Table"="", "Read Callback"="", "Write Callback"="", "Range Callback"="", "Check Callback"="", "Rngtable Callback"="", "Coerce Callback"="", "Supported Models"="", "Instrument Options"="", "Check Status Callback"="", "Flags"=0, "Help"="16-QAM / 64-QAM / 256-QAM modulation  limits definition."}, {"Level"=5, "Class Only"=FALSE, "Identifier"="RSCMXPNRFR2M_ATTR_MULTI_EVAL_MEASUREMENT_LIMIT_QAM16_EVM", "Descriptive Name"="Multi Eval Measurement Limit QAM16 EVM", "Data Type"=enum."RawString", "Command"="CONF:NRMM:MEAS{instance}:MEV:LIM:QAM16:EVM", "Access"=enum."Read/Write", "Range Table"="", "Read Callback"="", "Write Callback"="", "Range Callback"="", "Check Callback"="", "Rngtable Callback"="", "Coerce Callback"="", "Supported Models"="", "Instrument Options"="", "Check Status Callback"="", "Flags"=0, "Help"="Defines upper limits for the RMS and peak values of the error vector magnitude (EVM) for QAM16.\n\nSyntax:\nCONFigure:NRMMw:MEAS<i>:MEValuation:LIMit:QAM16:EVMagnitude <RMS>, <Peak>\n\n<RMS>\nnumeric | ON | OFF\nValid Values:\n0 % to 100 %\nOFF\nON\n  \n<Peak>\nnumeric | ON | OFF\nValid Values:\n0 % to 100 %\nOFF\nON\n\nAvailable Repeated Capabilities:\ninstance: i0, i1, i2, i3, i4, i5, i6, i7, i8, i9, i10, i11, i12, i13, i14, i15, i16, i17, i18, i19, i20, i21, i22, i23, i24, i25, i26, i27, i28, i29, i30, i31, i32\r\n\nRemote-control command(s):\nCONFigure:NRMMw:MEAS<i>:MEValuation:LIMit:QAM16:EVMagnitude"}, {"Level"=5, "Class Only"=FALSE, "Identifier"="RSCMXPNRFR2M_ATTR_MULTI_EVAL_MEASUREMENT_LIMIT_QAM64_EVM", "Descriptive Name"="Multi Eval Measurement Limit QAM64 EVM", "Data Type"=enum."RawString", "Command"="CONF:NRMM:MEAS{instance}:MEV:LIM:QAM64:EVM", "Access"=enum."Read/Write", "Range Table"="", "Read Callback"="", "Write Callback"="", "Range Callback"="", "Check Callback"="", "Rngtable Callback"="", "Coerce Callback"="", "Supported Models"="", "Instrument Options"="", "Check Status Callback"="", "Flags"=0, "Help"="Defines upper limits for the RMS and peak values of the error vector magnitude (EVM) for QAM64.\n\nSyntax:\nCONFigure:NRMMw:MEAS<i>:MEValuation:LIMit:QAM64:EVMagnitude <RMS>, <Peak>\n\n<RMS>\nnumeric | ON | OFF\nValid Values:\n0 % to 100 %\nOFF\nON\n  \n<Peak>\nnumeric | ON | OFF\nValid Values:\n0 % to 100 %\nOFF\nON\n\n
